vi "LockinDAQ.Start.AO.vi"(8 "error in (no error)":errorcluster, 11 "LockinDAQ":refnum<class "LockinDAQ.lvclass">) -> (0 "error out":errorcluster, 3 "LockinDAQ out":refnum<class "LockinDAQ.lvclass">)   [LabVIEW 2016, in "LockinDAQ.lvclass"]
uses:
  LockinDAQ.lvclass
  LockinDAQ.lvclass/LockinDAQ.ctl
  <vilib>/DAQmx/write.llb/DAQmx Write (Analog 1D Wfm NChan NSamp).vi
  <vilib>/DAQmx/miscellaneous.llb/DAQmx Fill In Error Info.vi
panel:
  out "reset indicator":bool
  out "Array":u32[](array[numeric])
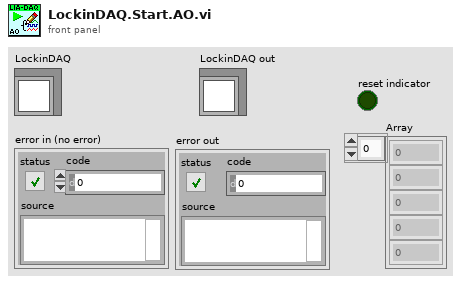
[diagram p1: front panel]
types:
  T1 = typedef "LockinDAQ.lvclass/AO-cluster.ctl" = cluster{"Ch":i32[], "Amp (V)":dbl[], "DC (V)":dbl[], "f (Hz)":dbl[], "Phase (°)":dbl[], "Function":T2[], "Sweep?":bool[]}
  T2 = typedef "LockinDAQ.lvclass/Function-enum.ctl" = enum16{"Sine", "Triangle", "Square", "Sawtooth"}
  T3 = typedef "LockinDAQ.lvclass/REF-cluster.ctl" = cluster{"Ch":i32[], " f (Hz)":dbl[], "Phase (°)":dbl[], "TC (s)":dbl[], "order":i32[]}
  T4 = typedef "LockinDAQ.lvclass/Sampling.ctl" = cluster{"Fs":dbl, "#s":i32}
  T5 = typedef "LockinDAQ.lvclass/DAQType-enum.ctl" = enum16{"None", "USB 4431", "PXI 446x"}
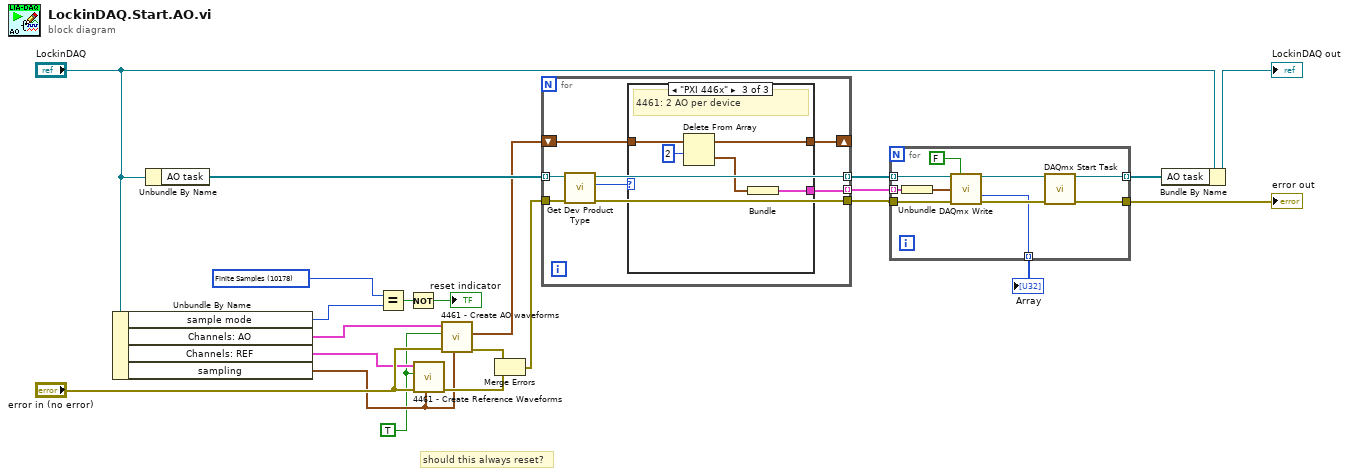
[diagram p0: block diagram]
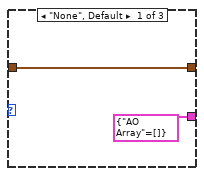
[diagram p2: hidden frame]
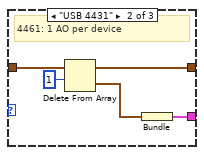
[diagram p3: hidden frame]
diagram:
  w1 = TRUE ("reset signal")
  w16 = 10178 items=["Finite Samples"=10178, "Continuous Samples"=10123] ("sample mode 2")
  # "should this always reset?"
  n1 = Unbundle By Name("LockinDAQ") -> ("sample mode"=w17:i32, "Channels: AO"=w19:T1, "Channels: REF"=w18:T3, "sampling"=w6:T4)
  n2 = Unbundle By Name("LockinDAQ") -> ("AO task"=w11:refnum<k21>[])
  n3 = Equal?(x=w16, y=w17) -> (x = y?=w20:bool)
  n4 = Not(x=w20) -> (.not. x?=→"reset indicator":bool)
  n5 = call "4461 - Create Reference Waveforms.vi"("sampling"=w6, "error in (no error)"="error in (no error)", "reset signal"=w1, "Lockin"=w18) -> ("error out"=w22:errorcluster)  [unwired: 4 in, 3 out]
  n6 = call "4461 - Create AO waveforms.vi"("sampling"=w6, "error in (no error)"="error in (no error)", "reset signal"=w1, "AO"=w19) -> ("error out"=w5:errorcluster, "AO Array"=w10:waveform(dbl)[])  [unwired: 4 in, 2 out]
  n7 = Merge Errors(w5, w22) -> (w4:errorcluster)
  n8 = for {
    tunnel: w11 -> [w30] mode=indexing
    shift-right: [w28] -> _
    shift-left: w10 -> [w29]
    tunnel: [w27] -> w9 mode=indexing
    tunnel: [w26] -> w8 mode=indexing
    tunnel: w4 -> [w25]
    tunnel: [w24] -> w7
    n9 = call "Get Dev Product Type.vi"("error in (no error)"=w25, "Refnum in"=w30) -> ("error out"=w24:errorcluster, "DAQ Type"=w23:T5, "Refnum out"=w26:refnum<k21>)  [unwired: 6 in, 1 out]
    n10 = case shown="\"PXI 446x\"" w23 {
      tunnel: w29 -> [w32 w37 w42]
      tunnel: [w32 w36 w41] -> w28
      tunnel: [cluster{"AO Array":waveform(dbl)[]} {"AO Array"=[]} w34 w38] -> w27
      frame "None", Default {
      }
      frame "USB 4431" {
        # "4461: 1 AO per device"
        n11 = Delete From Array(array=w37, length=1) -> (deleted portion=w33:waveform(dbl)[], array with subset deleted=w36:waveform(dbl)[])  [unwired: 1 in]
        n12 = Bundle("AO Array"=w33) -> (w34:cluster{"AO Array":waveform(dbl)[]})  [unwired: 1 in]
      }
      frame "PXI 446x" {
        # "4461: 2 AO per device"
        n13 = Delete From Array(array=w42, length=2) -> (deleted portion=w39:waveform(dbl)[], array with subset deleted=w41:waveform(dbl)[])  [unwired: 1 in]
        n14 = Bundle("AO Array"=w39) -> (w38:cluster{"AO Array":waveform(dbl)[]})  [unwired: 1 in]
      }
    }
  }
  n15 = for {
    tunnel: w8 -> [w50] mode=indexing
    tunnel: w7 -> [w49]
    tunnel: [w48] -> w12
    tunnel: [w47] -> w13 mode=indexing
    tunnel: w9 -> [w46] mode=indexing
    tunnel: [w43] -> w3 mode=indexing
    n16 = Unbundle(w46) -> ("AO Array"=w45:waveform(dbl)[])
    n17 = call-poly <vilib>:"DAQmx Write.vi"("task/channels in"=w50, "auto start"=FALSE, "data"=w45, "error in"=w49) -> ("task out"=w51:refnum<k21>, "number of samples written per channel"=w43:u32, "error out"=w52:errorcluster)  [unwired: 9 in]
    n18 = call <vilib>:"DAQmx Start Task.vi"("task/channels in"=w51, "error in"=w52) -> ("task out"=w47:refnum<k21>, "error out"=w48:errorcluster)  [unwired: 12 in]
  }
  "error out" <- w12
  "Array" <- w3
  n19 = Bundle By Name(cluster="LockinDAQ", "AO task"=w13) -> (→"LockinDAQ out":refnum<class "LockinDAQ.lvclass">)
